vi "global.vi"() -> ()   [LabVIEW 2018]
panel:
  in  "StringInput":string
  in  "NumericInput":dbl
  in  "ArrayString":string[](array[string])
  in  "ArrayNumber":dbl[](array[numeric])
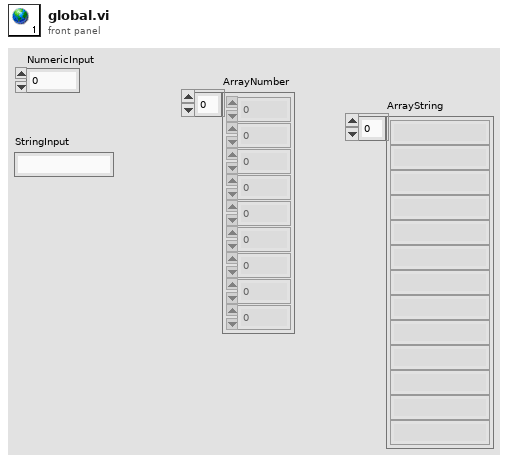
[diagram p1: front panel]
diagram:
